vi "Naughty VI Test.vi"   [LabVIEW 2024]
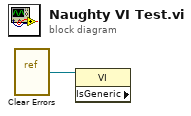
[diagram p0: block diagram]
diagram:
  n1 = vi-ref <vilib>:"Clear Errors.vi"() -> (w1:refnum<vi>)
  n2 = property class="VI" props=["IsGeneric"](reference=w1) -> ()  [unwired: 1 in, 3 out]
